vi "Coerce_Num.vi"(7 "Coerce towards +infinite?":bool, 10 "Num Step":i32=8, 11 "Num In":i32) -> (3 "Num Out":i32)   [LabVIEW 2019]
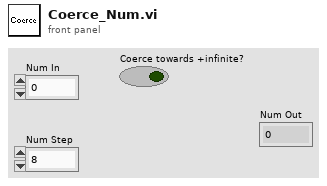
[diagram p1: front panel]
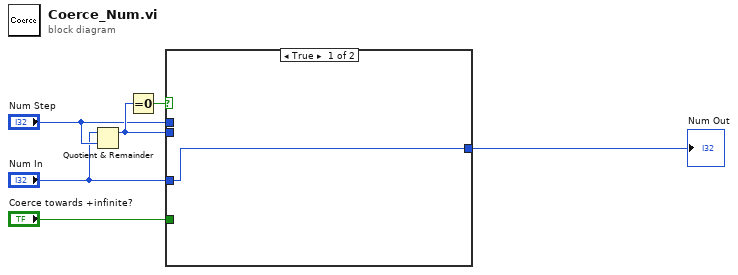
[diagram p0: block diagram]
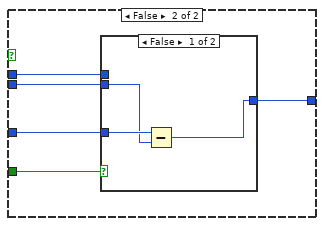
[diagram p2: hidden frame]
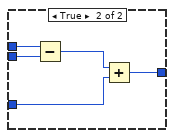
[diagram p3: hidden frame]
diagram:
  n1 = Quotient & Remainder(x="Num In", y="Num Step") -> (x-y*floor(x/y)=w6:i32)  [unwired: 1 out]
  n2 = Equal To 0?(x=w6) -> (x = 0?=w5:bool)
  n3 = case shown="True" w5 {
    tunnel: "Num Step" -> [_ w12]
    tunnel: w6 -> [_ w11]
    tunnel: "Coerce towards +infinite?" -> [_ w10]
    tunnel: "Num In" -> [w7 w9]
    tunnel: [w7 w8] -> w1
    frame True {
    }
    frame False {
      n4 = case shown="False" w10 {
        tunnel: w12 -> [_ w20]
        tunnel: w11 -> [w14 w19]
        tunnel: w9 -> [w15 w17]
        tunnel: [w13 w16] -> w8
        frame False {
          n5 = Subtract(x=w15, y=w14) -> (x-y=w13:i32)
        }
        frame True {
          n6 = Subtract(x=w20, y=w19) -> (x-y=w18:i32)
          n7 = Add(x=w18, y=w17) -> (x+y=w16:i32)
        }
      }
    }
  }
  "Num Out" <- w1
